vi "Reset all components.vi"(8 "error in (no error)":errorcluster, 11 "Panel in":refnum<class "Station Actor.lvclass">) -> (0 "error out":errorcluster, 3 "Panel out":refnum<class "Station Actor.lvclass">)   [LabVIEW 2019, in "Station Actor.lvlib" / "Station Actor.lvclass"]
uses:
  Station Actor.lvclass
  Station Actor.lvclass/Station Actor.ctl
  Custom Controls/Tester Rx Dataset.ctl
  Custom Controls/Tester Tx Dataset.ctl
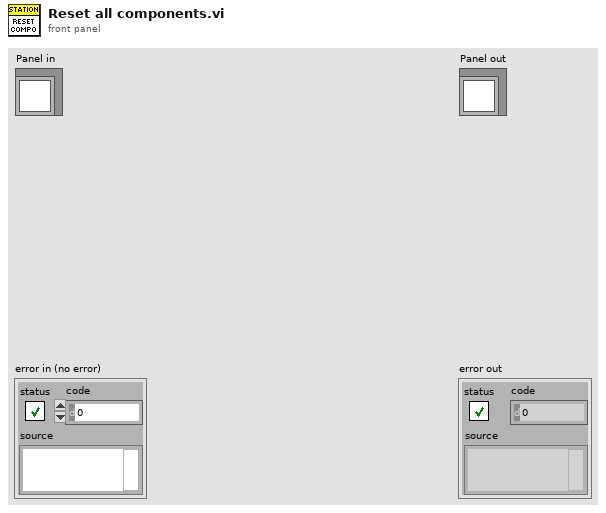
[diagram p1: front panel]
types:
  T1 = typedef "Station Actor.lvlib/Station Actor.lvclass/Tester Tx Dataset.ctl" = cluster{"Fault":bool, "StepNo":u32, "Ready":bool, "HighVoltage":bool, "TestRunning":bool, "ResultsReady":bool, "Results":u32, "ElapsedTime":u32, "Online":bool, "TimeCompleted":i32[], "Timeout":bool, "Heartbeat":bool}
  T2 = typedef "Station Actor.lvlib/Station Actor.lvclass/Tester Rx Dataset.ctl" = cluster{"Start":bool, "NestStatus":bool, "PalletID":u32, "BarcodeData":string, "StepEcho":u32, "Cylinder_1":bool, "Cylinder_2":bool, "Cylinder_3":bool, "Cylinder_4":bool, "Cylinder_5":bool, "ResultsAck":bool, "Reset":bool, "Stop":bool, "FaultCode":u32}
  T3 = typedef "Panel.lvlib/Panel.lvclass/Tester Tx Dataset.ctl" = cluster{"Fault":bool, "StepNo":u32, "Ready":bool, "HighVoltage":bool, "TestRunning":bool, "ResultsReady":bool, "Results":u32, "ElapsedTime":u32, "Online":bool, "TimeCompleted":i32[], "Timeout":bool, "Heartbeat":bool}
  T4 = typedef "Panel.lvlib/Panel.lvclass/Tester Rx Dataset.ctl" = cluster{"Start":bool, "NestStatus":bool, "PalletID":u32, "BarcodeData":string, "StepEcho":u32, "Cylinder_1":bool, "Cylinder_2":bool, "Cylinder_3":bool, "Cylinder_4":bool, "Cylinder_5":bool, "ResultsAck":bool, "Reset":bool, "Stop":bool, "FaultCode":u32}
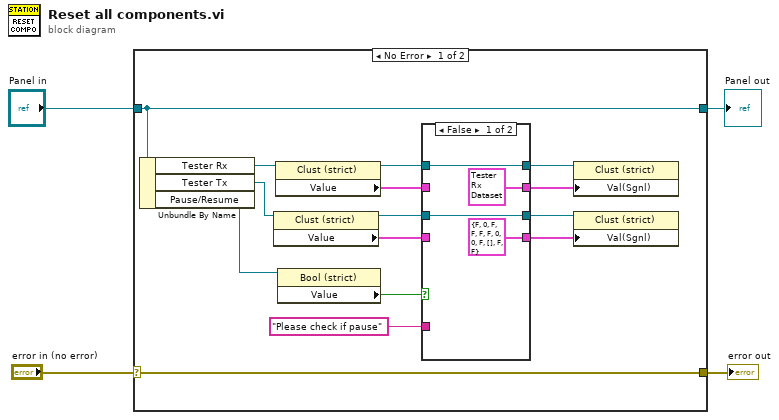
[diagram p0: block diagram]
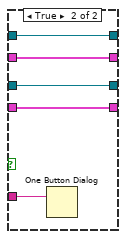
[diagram p2: hidden frame]
diagram:
  n1 = case shown="No Error" "error in (no error)" {
    selector: "error in (no error)" -> [w19 w30]
    tunnel: [w19 w30] -> w3
    tunnel: [w18 w29] -> w1
    tunnel: "Panel in" -> [w18 w29]
    frame No Error {
      n2 = Unbundle By Name(w18) -> ("Tester Rx"=w17:refnum<vi>, "Tester Tx"=w11:refnum<vi>, "Pause/Resume"=w16:refnum<vi>)
      n3 = property class="Clust (strict)"(reference=w11) -> (reference out=w8:refnum<vi>, "Value"=w6:T3)  [unwired: 1 in, 1 out]
      n4 = property class="Clust (strict)"(reference=w17) -> (reference out=w10:refnum<vi>, "Value"=w13:T4)  [unwired: 1 in, 1 out]
      n5 = property class="Bool (strict)"(reference=w16) -> ("Value"=w15:bool)  [unwired: 1 in, 2 out]
      n6 = case shown="False" w15 {
        tunnel: [T2 {"Start"=FALSE, "NestStatus"=FALSE, "PalletID"=0, "BarcodeData"="P:10-000001R:04S:QMC2200001", "StepEcho"=0, "Cylinder_1"=FALSE, "Cylinder_2"=FALSE, "Cylinder_3"=FALSE, "Cylinder_4"=FALSE, "Cylinder_5"=FALSE, "ResultsAck"=FALSE, "Reset"=FALSE, "Stop"=FALSE, "FaultCode"=0} ("Rx from PLC") w28] -> w14
        tunnel: w13 -> [_ w28]
        tunnel: "Please check if pause" ("message") -> [_ w27]
        tunnel: w10 -> [w23 w26]
        tunnel: [w23 w26] -> w9
        tunnel: w8 -> [w22 w25]
        tunnel: [w22 w25] -> w7
        tunnel: w6 -> [_ w24]
        tunnel: [T1 {"Fault"=FALSE, "StepNo"=0, "Ready"=FALSE, "HighVoltage"=FALSE, "TestRunning"=FALSE, "ResultsReady"=FALSE, "Results"=0, "ElapsedTime"=0, "Online"=FALSE, "TimeCompleted"=[], "Timeout"=FALSE, "Heartbeat"=FALSE} ("Tx to PLC") w24] -> w5
        frame False {
        }
        frame True {
          n7 = One Button Dialog(message=w27) -> ()  [unwired: 1 in, 1 out]
        }
      }
      n8 = property class="Clust (strict)"(reference=w9, "Val(Sgnl)"=w14) -> ()  [unwired: 1 in, 2 out]
      n9 = property class="Clust (strict)"(reference=w7, "Val(Sgnl)"=w5) -> ()  [unwired: 1 in, 2 out]
    }
    frame Error {
    }
  }
  "error out" <- w3
  "Panel out" <- w1
